vi "Generate indices and data.vi"(7 "Length":i32, 11 "Sample size":i32) -> (2 "Data":dbl[](array[numeric]), 3 "Indices":u32[](array[numeric]))   [LabVIEW 2018]
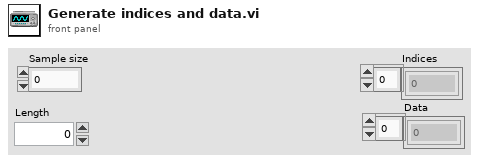
[diagram p1: front panel]
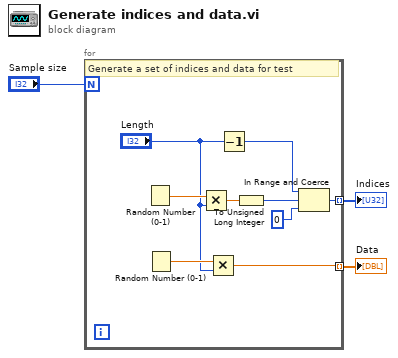
[diagram p0: block diagram]
diagram:
  n1 = for {
    N: "Sample size" -> [_]
    tunnel: [w9] -> w2 mode=indexing
    tunnel: [w7] -> w3 mode=indexing
    # "Generate a set of indices and data for test"
    n2 = Random Number (0-1)() -> (number: 0 to 1=w12:dbl)
    n3 = Random Number (0-1)() -> (number: 0 to 1=w10:dbl)
    n4 = Multiply(x=w12, y="Length") -> (x*y=w11:dbl)
    n5 = Multiply(x=w10, y="Length") -> (x*y=w9:dbl)
    n6 = Decrement(x="Length") -> (x-1=w4:i32)
    n7 = To Unsigned Long Integer(number=w11) -> (unsigned 32bit integer=w8:u32)
    n8 = In Range and Coerce(upper limit=w4, x=w8, lower limit=u32 0) -> (coerced(x)=w7:u32)  [unwired: 1 out]
  }
  "Indices" <- w3
  "Data" <- w2
